vi "thermo_get_result_means.vi"(2 "temp channel":T1[][](array[typedef])) -> (1 "pressure":dbl format="%0.2f", 4 "pres vector":dbl[](array[numeric]), 5 "RH":dbl format="%0.2f", 6 "temp":dbl format="%0.2f", 7 "N":i32, 8 "RH vector":dbl[](array[numeric]), 9 "temp vector":dbl[](array[numeric]))   [LabVIEW 2020]
uses:
  thermo_read.ctl
  <vilib>/Analysis/baseanly.llb/Mean (DBL).vi
  <vilib>/Analysis/NI_AALBase.lvlib
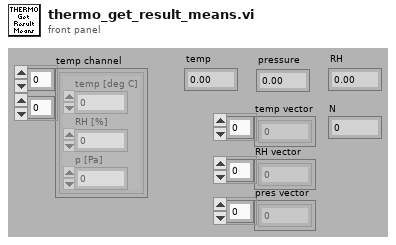
[diagram p1: front panel]
types:
  T1 = typedef "thermo_read.ctl" = cluster{"temp [deg C]":dbl, "RH [%]":dbl, "p [Pa]":dbl}
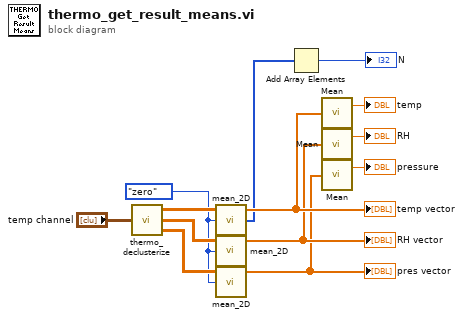
[diagram p0: block diagram]
diagram:
  w1 = enum16{"none", "invalids", "zero"}."zero" ("filter")
  n1 = call "thermo_declusterize.vi"("temp channel"="temp channel") -> ("temperature"=w4:dbl[][], "RH"=w12:dbl[][], "pressure"=w11:dbl[][])
  n2 = call "mean_2D.vi"("filter"=w1, "2D array"=w4) -> ("counts"=w3:i32[], "means"=w10:dbl[])  [unwired: 1 in, 1 out]
  "temp vector" <- w10
  n3 = call "mean_2D.vi"("filter"=w1, "2D array"=w12) -> ("means"=w6:dbl[])  [unwired: 1 in, 2 out]
  "RH vector" <- w6
  n4 = call "mean_2D.vi"("filter"=w1, "2D array"=w11) -> ("means"=w5:dbl[])  [unwired: 1 in, 2 out]
  "pres vector" <- w5
  n5 = Add Array Elements(numeric array=w3) -> (sum=→"N":i32)
  n6 = call-poly <vilib>:"Mean.vi"("X"=w10) -> ("mean"=→"temp":dbl)  [unwired: 1 out]
  n7 = call-poly <vilib>:"Mean.vi"("X"=w6) -> ("mean"=→"RH":dbl)  [unwired: 1 out]
  n8 = call-poly <vilib>:"Mean.vi"("X"=w5) -> ("mean"=→"pressure":dbl)  [unwired: 1 out]
